vi "Sparse - Scale Nodes Linear.vi"(8 "error in (no error)":errorcluster, 9 "Scaling limits":cluster{"X lower":dbl, "X upper":dbl}, 10 "xmaxmin":cluster{"min":dbl, "max":dbl}[](array[cluster]), 11 "x":T1[](array[typedef])) -> (0 "error out":errorcluster, 3 "x scaled":T1[](array[typedef]))   [LabVIEW 2014]
uses:
  LibSVM Sparse/Wrapper API/Controls/svm_node.ctl
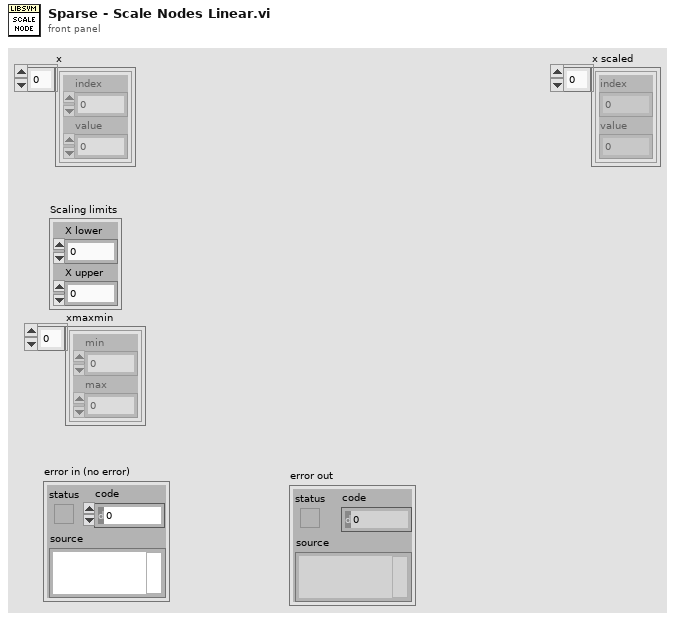
[diagram p1: front panel]
types:
  T1 = typedef "svm_node.ctl" = cluster{"index":i32, "value":dbl}
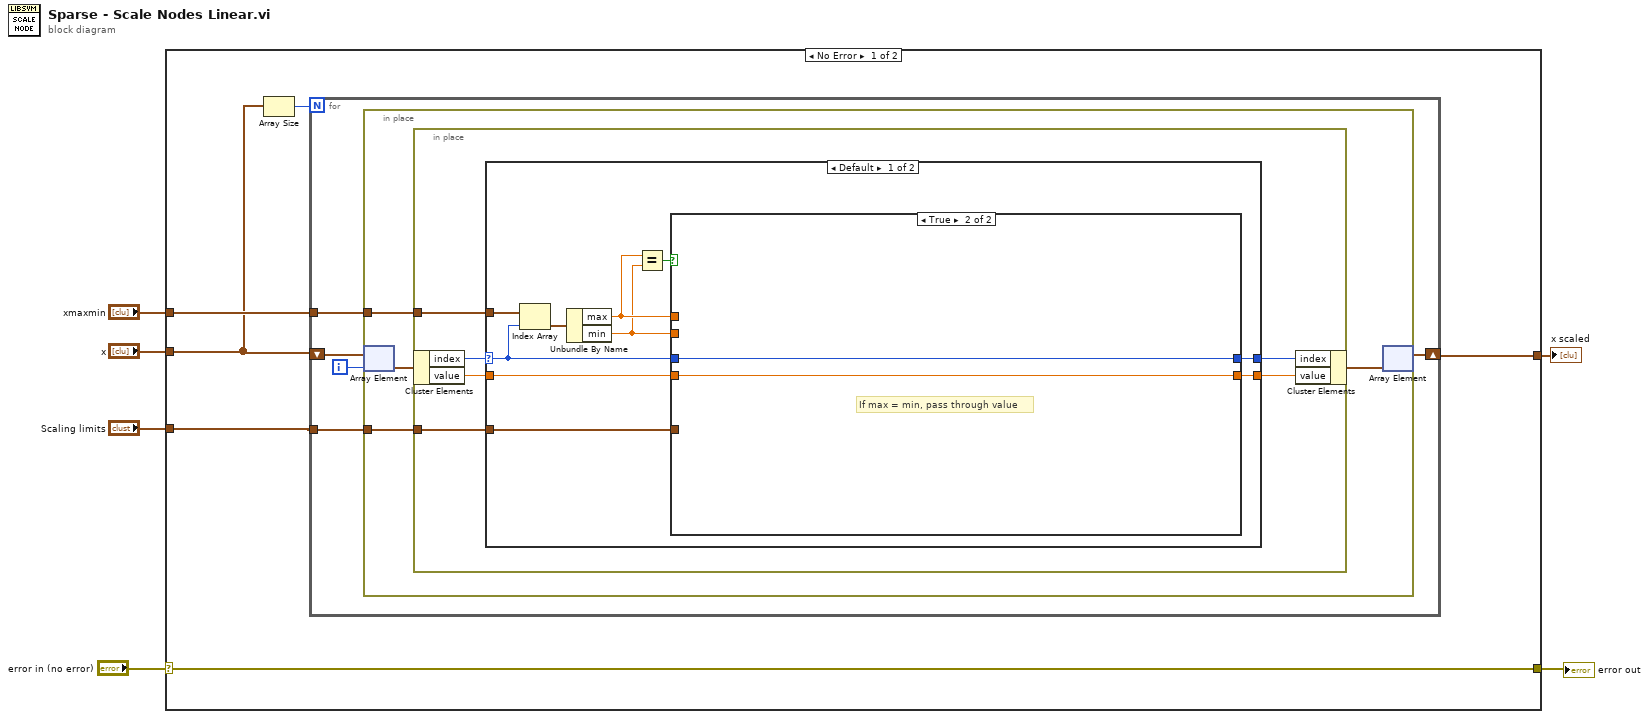
[diagram p0: block diagram]
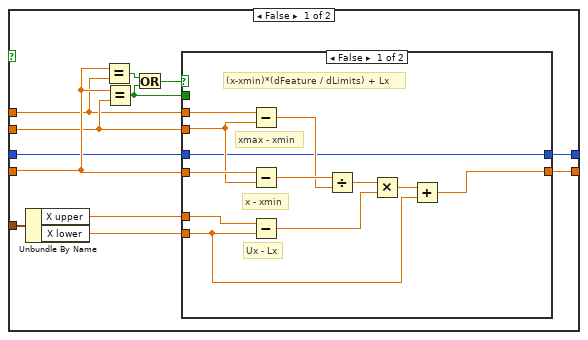
[diagram p2: hidden frame]
diagram:
  n1 = case shown="No Error" "error in (no error)" {
    selector: "error in (no error)" -> [w10 w76]
    tunnel: [w10 w76] -> w6
    tunnel: "Scaling limits" -> [w12 _]
    tunnel: "xmaxmin" -> [w11 _]
    tunnel: [w8 _] -> w2
    tunnel: "x" -> [w7 _]
    frame No Error {
      n2 = Array Size(array=w7) -> (size(s)=w9:i32)
      n3 = for {
        N: w9 -> [_]
        shift-right: [w16] -> w8
        shift-left: w7 -> [w17]
        tunnel: w11 -> [w15]
        tunnel: w12 -> [w14]
        i -> [w13]
        n4 = in-place {
          in-place-border: w15 -> [w21]
          in-place-border: w14 -> [w20]
          n5 = in-place-array #1(w17, w13) -> (w19:T1)
          n6 = in-place {
            in-place-border: w21 -> [w27]
            in-place-border: w20 -> [w26]
            n7 = in-place-cluster #2(w19) -> ("index"=w25:i32, "value"=w24:dbl)
            n8 = case shown="Default" w25 {
              selector: w25 -> [w31 w75]
              tunnel: w24 -> [w32 w74]
              tunnel: w27 -> [w37 _]
              tunnel: w26 -> [w30 _]
              tunnel: [w29 w74] -> w23
              tunnel: [w28 w75] -> w22
              frame Default {
                n9 = Index Array(array=w37, index=w31) -> (element=w36:cluster{"min":dbl, "max":dbl})
                n10 = Unbundle By Name(w36) -> ("max"=w34:dbl, "min"=w33:dbl)
                n11 = Equal?(x=w34, y=w33) -> (x = y?=w35:bool)
                n12 = case shown="True" w35 {
                  tunnel: w34 -> [w44 _]
                  tunnel: w33 -> [w45 _]
                  tunnel: w32 -> [w46 w72]
                  tunnel: w31 -> [w38 w73]
                  tunnel: w30 -> [w49 _]
                  tunnel: [w40 w72] -> w29
                  tunnel: [w39 w73] -> w28
                  frame False {
                    # "maxmin not equal"
                    n13 = Unbundle By Name(w49) -> ("X upper"=w42:dbl, "X lower"=w41:dbl)
                    n14 = Equal?(x=w46, y=w44) -> (x = y?=w48:bool)
                    n15 = Equal?(x=w46, y=w45) -> (x = y?=w43:bool)
                    n16 = Or(x=w48, y=w43) -> (x .or. y?=w47:bool)
                    n17 = case shown="False" w47 {
                      tunnel: w46 -> [w60 _]
                      tunnel: w44 -> [w59 _]
                      tunnel: w45 -> [w58 _]
                      tunnel: w43 -> [_ w67]
                      tunnel: w42 -> [w61 w66]
                      tunnel: w41 -> [w52 w65]
                      tunnel: [w51 w64] -> w40
                      tunnel: [w50 w63] -> w39
                      tunnel: w38 -> [w50 w62]
                      frame False {
                        # "(x-xmin)*(dFeature / dLimits) + Lx"
                        # "xmax - xmin"
                        # "x - xmin"
                        # "Ux - Lx"
                        n18 = Subtract(x=w59, y=w58) -> (x-y=w56:dbl)
                        n19 = Subtract(x=w60, y=w58) -> (x-y=w57:dbl)
                        n20 = Subtract(x=w61, y=w52) -> (x-y=w54:dbl)
                        n21 = Divide(x=w57, y=w56) -> (x/y=w55:dbl)
                        n22 = Multiply(x=w55, y=w54) -> (x*y=w53:dbl)
                        n23 = Add(x=w53, y=w52) -> (x+y=w51:dbl)
                      }
                      frame True {
                        n24 = case shown="False" w67 {
                          tunnel: w66 -> [w69 _]
                          tunnel: w65 -> [_ w71]
                          tunnel: [w69 w71] -> w64
                          tunnel: [w68 w70] -> w63
                          tunnel: w62 -> [w68 w70]
                          frame False {
                          }
                          frame True {
                          }
                        }
                      }
                    }
                  }
                  frame True {
                    # "If max = min, pass through value"
                    # "set to"
                  }
                }
              }
              frame -1 {
              }
            }
            n25 = in-place-cluster #2("index"=w22, "value"=w23) -> (w18:T1)
          }
          n26 = in-place-array #1(w18) -> (w16:T1[])  [unwired: 1 out]
        }
      }
    }
    frame Error {
    }
  }
  "error out" <- w6
  "x scaled" <- w2
